vi "Main myRIO.vi"() -> ()   [LabVIEW 2012]
uses:
  <vilib>/rvi/interface/nirviOpenFPGA/nirviOpenFPGA.xnode
  FPGA Bitfiles/PDMSrobotcode_FPGATarget_AllIOs_I1UhDttAVn8.lvbitx
  FPGA/All IOs.vi
  <vilib>/FPGAPlugInAG/myRIO-1900/niLvFpga_Open_myRIO-1900.vi
  <vilib>/rvi/interface/common/dynamic/niFpgaDynamicAddResources.vi
  <vilib>/rvi/interface/nirviReadWriteControl/nirviReadWriteControl.xnode
  <vilib>/rvi/interface/Simulation/niFpgaSimulationCallBeginRW.vi
  <vilib>/rvi/errors/niLvFpgaAdjustHostInterfaceError.vi
  NiFpgaLv.dll
  <vilib>/Utility/error.llb/Error Cluster From Error Code.vi
  <vilib>/rvi/interface/nirviCloseFPGA/nirviCloseFPGA.xnode
  <vilib>/FPGAPlugInAG/Dynamic/niLvFpga_Close_Dynamic.vi
  <vilib>/myRIO/Instrument Drivers/Utilities/Utilities.lvlib
  <vilib>/Instr/_visa.llb/VISA Configure Serial Port (Instr).vi
  <vilib>/myRIO/Instrument Drivers/Onboard IO/UART/typedef/VISA Configuration.ctl
  <vilib>/myRIO/Instrument Drivers/Onboard IO/UART/UART.lvlib
panel:
  in  "Standalone?":bool
  out "BMP180 Data":string
  out "NMEA sentences":string
  out "Time":string
  in  "time zone":i32
  out "Latitude [deg]":string
  out "Longitude [deg]":string
  out "UTC Time":string
  out "Latitude":string
  out "N/S":string
  out "Longitude":string
  out "E/W":string
  out "Speed over ground [knots]":string
  out "Status":string
  out "Course over ground [degrees]":string
  out "Date [ddmmyy]":string
  out "Mode":string
  in  "Acquire?":bool
  out "Frame Rate":dbl
  out "Image Number":u32
  in  "Capture":bool
  in  "Image Logging path":path
  out "Image":T1(plugin-control)
  in  "Down Button":bool
  in  "Left Button":bool
  out "Distance in cm (US BK)":i16
  out "Distance in cm (US FR)":i16
  out "Distance in cm (US FL)":i16
  out "Error":errorcluster
  out "IR Sensors":T2
  in  "Robotic Arm Controls":T3
  in  "Stop Button":bool
  in  "Right Button":bool caption="Next Button"
  in  "Up Button":bool
  out "Inclination":T4(graph)
  # "LED Brightnesses"
  # "GPS Data"
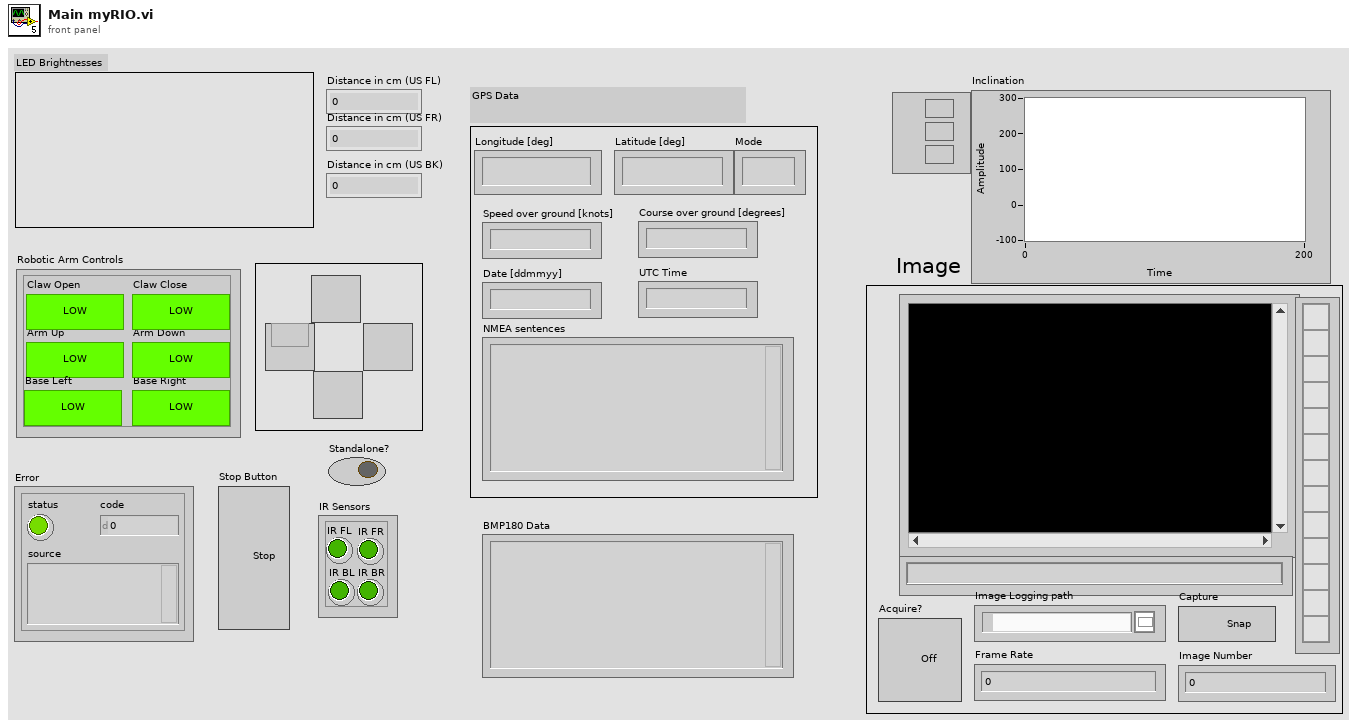
[diagram p1: front panel]
types:
  T1 = typedef "IMAQ Image.ctl" = refnum<image>
  T2 = cluster{"IR FL":bool, "IR FR":bool, "IR BR":bool, "IR BL":bool}
  T3 = cluster{"Arm Up":bool, "Claw Open":bool, "Base Right":bool, "Arm Down":bool, "Base Left":bool, "Claw Close":bool}
  T4 = cluster{"AccelerationX":i16, "AccelerationY":i16, "AccelerationZ":i16}
  T5 = cluster{"Time of flight (uS) (US FL)":u32, "Time of flight (uS) (US FR)":u32, "Time of flight (uS) (US BK)":u32}
  T6 = cluster{"UP":bool, "DOWN":bool, "LEFT":bool, "RIGHT":bool}
  T7 = typedef "UART.lvlib/VISA Configuration.ctl" = cluster{"baud rate (9600)":u32, "data bits (8)":u16, "parity (0:none)":enum16{"None", "Odd", "Even", "Mark", "Space"}, "stop bits (10: 1 bit)":u16, "flow control (0:none)":u16, "termination char\n(0xA = '\\n' = LF) ":u8, "Enable Termination\nChar (T)":bool, "timeout (10sec)":u32}
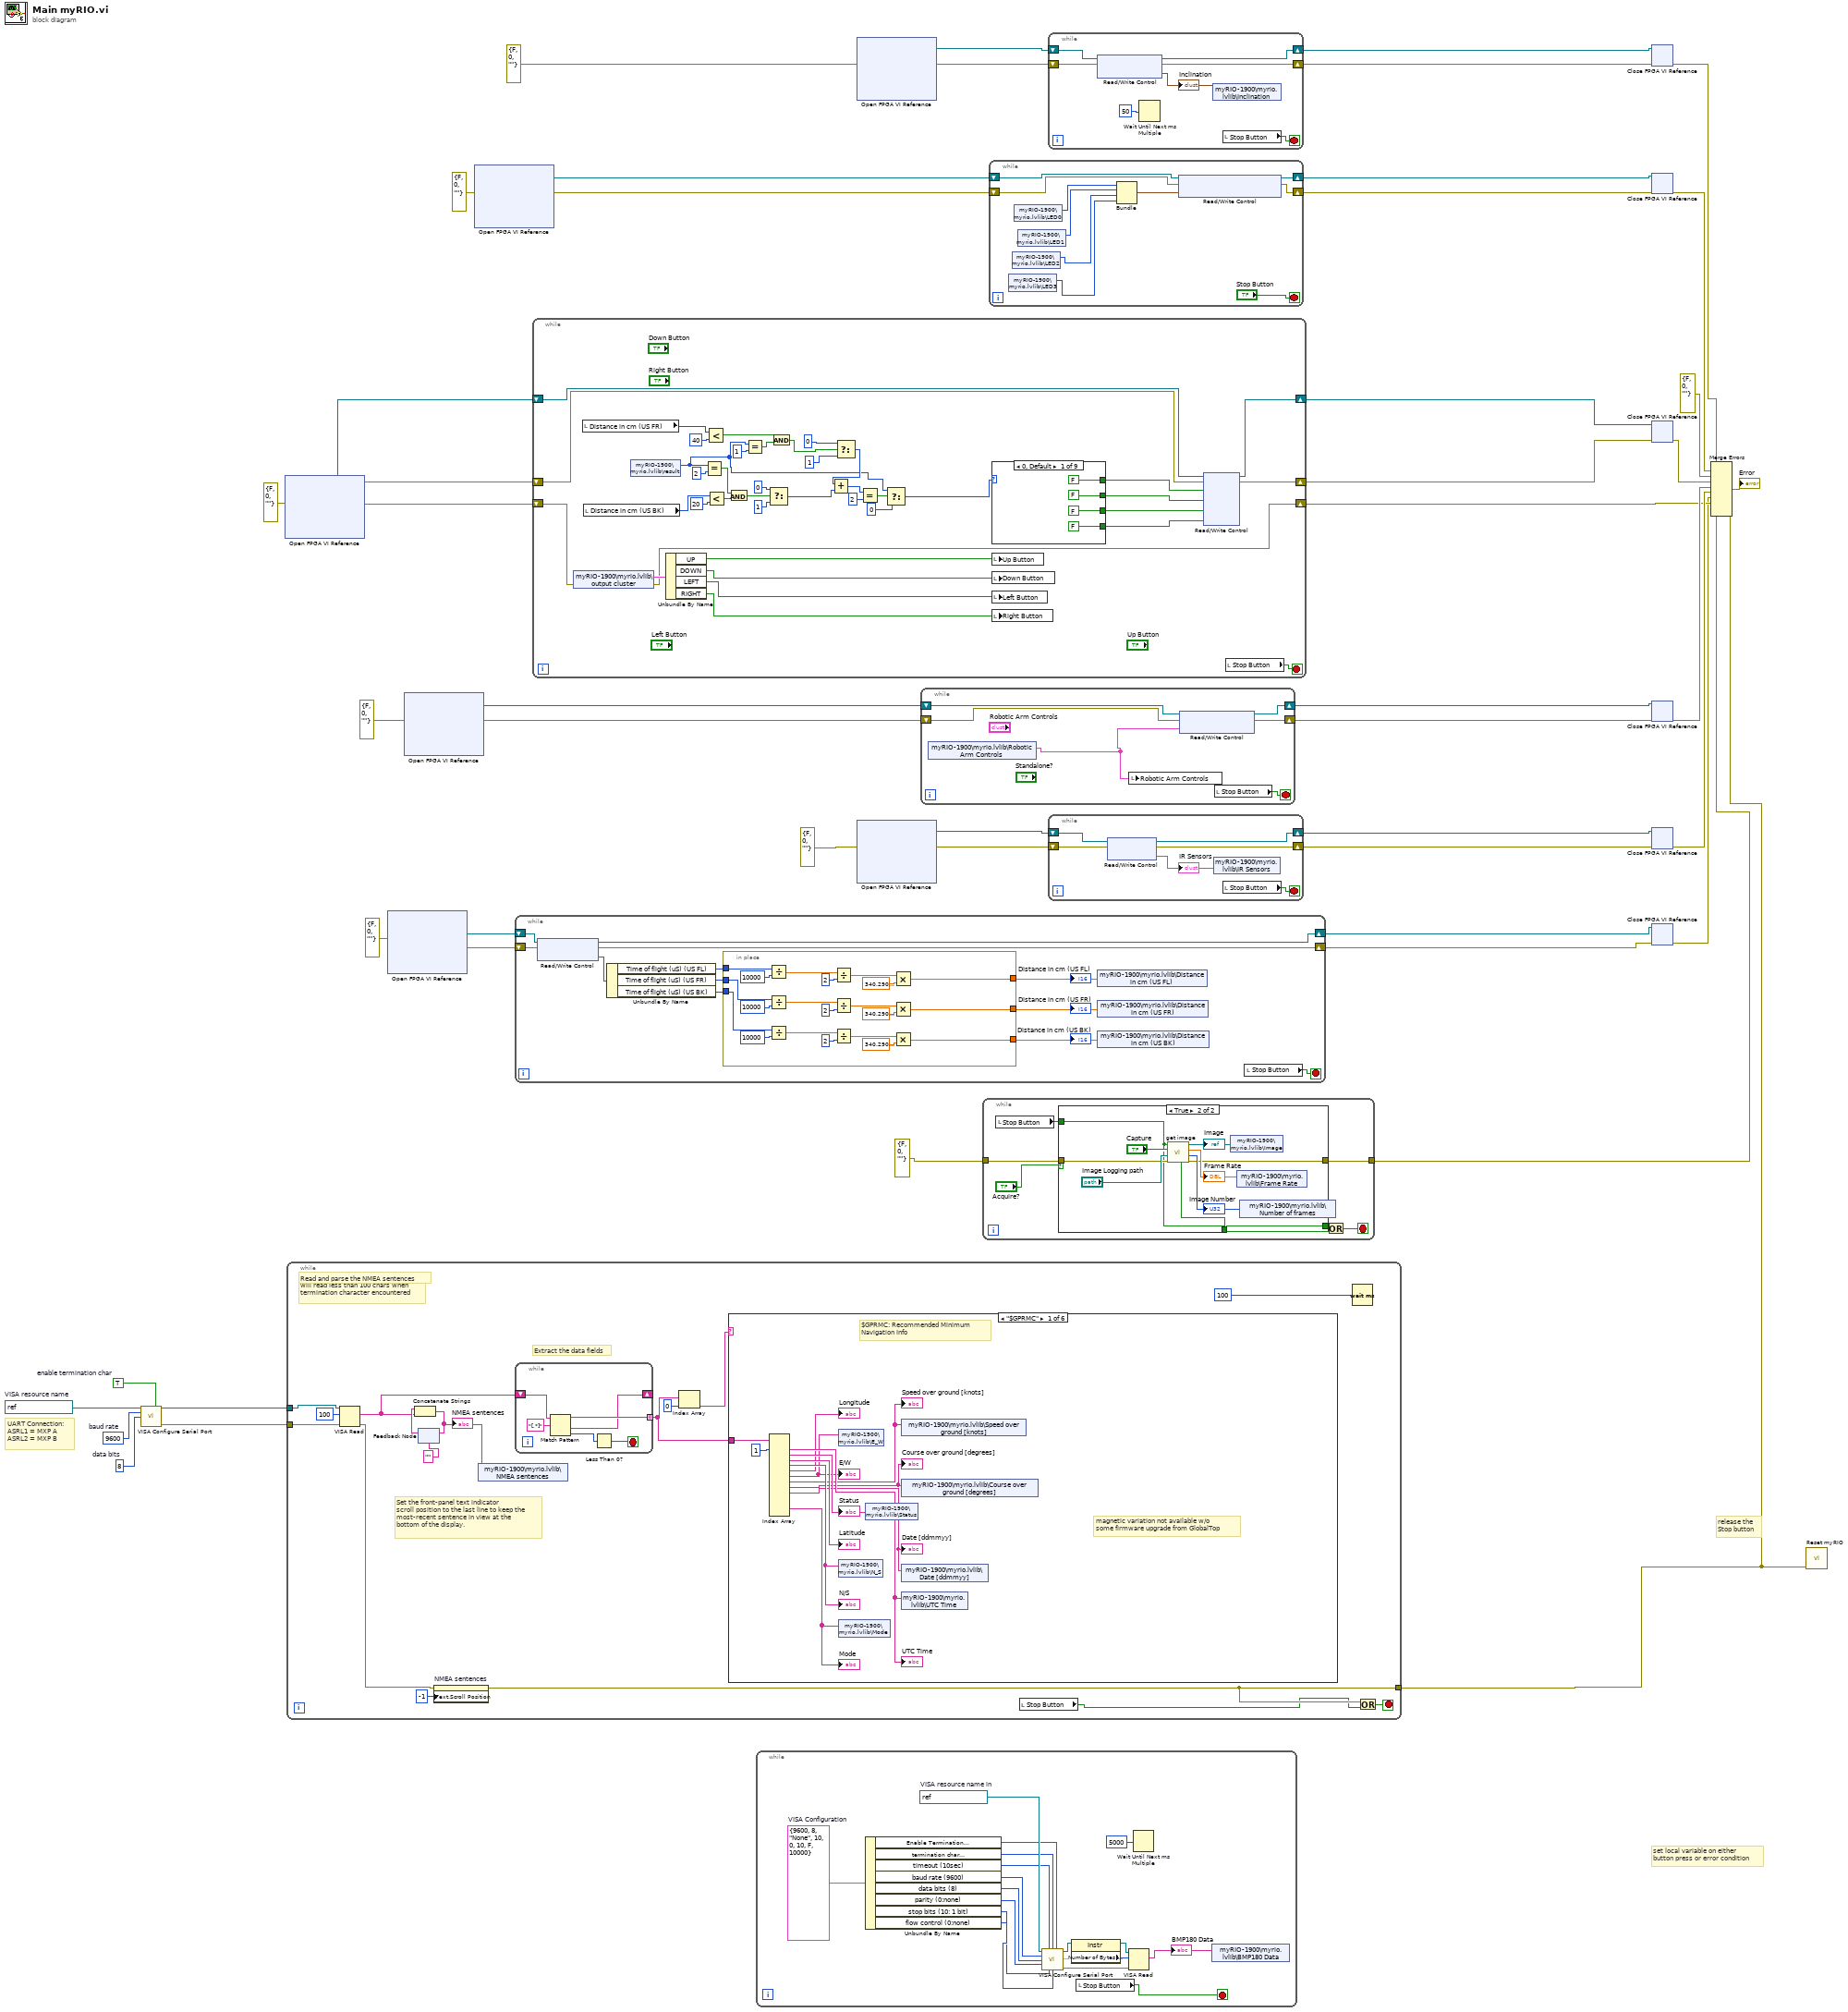
[diagram p0: block diagram]
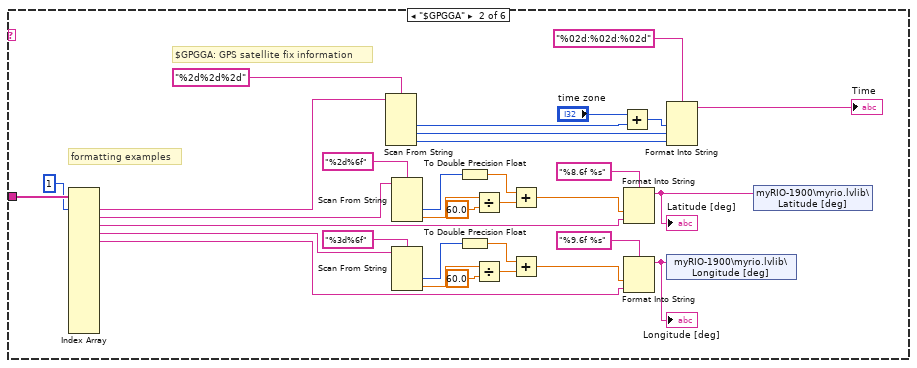
[diagram p2: hidden frame]
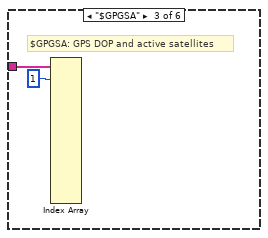
[diagram p3: hidden frame]
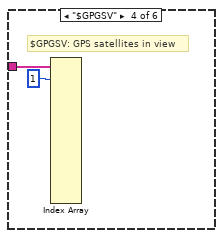
[diagram p4: hidden frame]
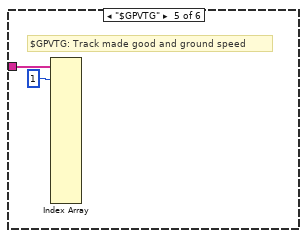
[diagram p5: hidden frame]
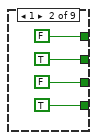
[diagram p8: hidden frame]
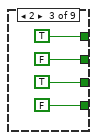
[diagram p9: hidden frame]
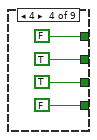
[diagram p10: hidden frame]
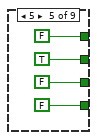
[diagram p11: hidden frame]
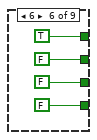
[diagram p12: hidden frame]
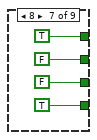
[diagram p13: hidden frame]
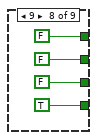
[diagram p14: hidden frame]
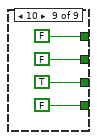
[diagram p15: hidden frame]
diagram:
  w4 = TRUE  # enable termination char
  w5 = u16 8  # data bits
  w6 = u32 9600  # baud rate
  w8 = refnum<visa-resource-name> "ASRL2::INSTR"  # VISA resource name
  # "release the\nStop button"
  # "set local variable on either\nbutton press or error condition"
  # "UART Connection:\nASRL1 = MXP A \nASRL2 = MXP B"
  n1 = call-poly "VISA Configure Serial Port"("VISA resource name"=w8, "Enable Termination\nChar (T)"=w4, "baud rate (9600)"=w6, "data bits (8)"=w5) -> ("VISA resource name out"=w7:refnum<visa-resource-name>, "error out"=w3:errorcluster)  [unwired: 10 in]
  n2 = xnode "Open FPGA VI Reference"("error in"=errorcluster {"status"=FALSE, "code"=0, "source"=""}) -> ("FPGA VI Reference Out"=w35:refnum<k20>, "error out"=w14:errorcluster)  [unwired: 1 in]
  n3 = while {
    tunnel: [w51] -> w2
    tunnel: w7 -> [w63]
    tunnel: w3 -> [w57]
    stop <- w50 stop-if-true
    # "Set the front-panel text indicator\nscroll position to the last line to keep the\nmost-recent sentence in view at the\nbottom of the display."
    # "Read and parse the NMEA sentences"
    # "Extract the data fields"
    # "Read a complete sentence;\nwill read less than 100 chars when\ntermination character encountered"
    n4 = VISA Read(VISA resource name=w63, byte count=u32 100, error in (no error)=w57) -> (read buffer=w58:string, error out=w52:errorcluster)  [unwired: 2 out]
    n5 = feedback #1("") -> (w60:string)
    n6 = Concatenate Strings "Concatenate Strings"(w60, w58) -> (w62:string)
    "NMEA sentences" <- w62
    n7 = feedback-in #1(w62) -> ()
    n8 = property on="NMEA sentences" class="Str"(error in=w52, "Text.Scroll Position"=-1) -> (error out=w51:errorcluster)  [unwired: 1 in, 1 out]
    n9 = shared-variable "myRIO-1900\\myrio.lvlib\\NMEA sentences"(w62) -> ()  [unwired: 1 in, 1 out]
    n10 = while {
      tunnel: [w119] -> w55 mode=indexing
      shift-right: [w118] -> _
      shift-left: w58 -> [w120]
      stop <- w117 stop-if-true
      n11 = Match Pattern(string=w120, regular expression="[,*]") -> (before substring=w119:string, after substring=w118:string, offset past match=w116:i32)  [unwired: 1 in, 1 out]
      n12 = Less Than 0?(x=w116) -> (x < 0?=w117:bool)
    }
    n13 = Index Array "Index Array"(array=w55, index=0) -> (element=w56:string)
    n14 = case shown="\"$GPRMC\"" w56 {
      tunnel: w55 -> [w76 w109 w111 w113 w115 _]
      frame "$GPRMC" {
        # "magnetic variation not available w/o\nsome firmware upgrade from GlobalTop"
        # "$GPRMC: Recommended Minimum\nNavigation Info"
        n15 = Index Array "Index Array"(array=w76, index #1=1 ("index")) -> (element #1=w75:string, element #2=w73:string, element #3=→"Latitude":string, element #4=w71:string, element #5=→"Longitude":string, element #6=w69:string, element #7=w67:string, element #8=w65:string, element #9=w66:string, element #12=w68:string)  [unwired: 12 in, 3 out]
        "UTC Time" <- w75
        "N/S" <- w71
        "E/W" <- w69
        "Speed over ground [knots]" <- w67
        "Status" <- w73
        "Course over ground [degrees]" <- w65
        "Date [ddmmyy]" <- w66
        "Mode" <- w68
        n16 = shared-variable "myRIO-1900\\myrio.lvlib\\E_W"(w69) -> ()  [unwired: 1 in, 1 out]
        n17 = shared-variable "myRIO-1900\\myrio.lvlib\\N_S"(w71) -> ()  [unwired: 1 in, 1 out]
        n18 = shared-variable "myRIO-1900\\myrio.lvlib\\Mode"(w68) -> ()  [unwired: 1 in, 1 out]
        n19 = shared-variable "myRIO-1900\\myrio.lvlib\\Status"(w73) -> ()  [unwired: 1 in, 1 out]
        n20 = shared-variable "myRIO-1900\\myrio.lvlib\\Speed over ground [knots]"(w67) -> ()  [unwired: 1 in, 1 out]
        n21 = shared-variable "myRIO-1900\\myrio.lvlib\\Course over ground [degrees]"(w65) -> ()  [unwired: 1 in, 1 out]
        n22 = shared-variable "myRIO-1900\\myrio.lvlib\\Date [ddmmyy]"(w66) -> ()  [unwired: 1 in, 1 out]
        n23 = shared-variable "myRIO-1900\\myrio.lvlib\\UTC Time"(w75) -> ()  [unwired: 1 in, 1 out]
      }
      frame "$GPGGA" {
        # "formatting examples"
        # "$GPGGA: GPS satellite fix information"
        n24 = Index Array "Index Array"(array=w109, index #1=1 ("index")) -> (element #1=w106:string, element #2=w97:string, element #3=w89:string, element #4=w78:string, element #5=w77:string)  [unwired: 15 in, 11 out]
        n25 = Scan From String "Scan From String"(format string="%2d%2d%2d", input string=w106) -> (output 1=w99:i32, output 2=w102:i32, output 3=w104:i32)  [unwired: 5 in, 3 out]
        n26 = Scan From String(format string="%2d%6f", input string=w97) -> (output 1=w94:i32, output 2=w96:dbl)  [unwired: 4 in, 3 out]
        n27 = Scan From String(format string="%3d%6f", input string=w78) -> (output 1=w82:i32, output 2=w80:dbl)  [unwired: 4 in, 3 out]
        n28 = To Double Precision Float(number=w94) -> (double precision float=w92:dbl)
        n29 = To Double Precision Float(number=w82) -> (double precision float=w84:dbl)
        n30 = Divide(x=w96, y=60.0) -> (x/y=w93:dbl)
        n31 = Divide(x=w80, y=60.0) -> (x/y=w83:dbl)
        n32 = Add(x=w92, y=w93) -> (x+y=w90:dbl)
        n33 = Add(x=w84, y=w83) -> (x+y=w86:dbl)
        n34 = Add(x="time zone", y=w99) -> (x+y=w100:i32)
        n35 = Format Into String(format string="%8.6f %s", w90, w89) -> (resulting string=w88:string)  [unwired: 2 in, 1 out]
        "Latitude [deg]" <- w88
        n36 = Format Into String(format string="%9.6f %s", w86, w77) -> (resulting string=w87:string)  [unwired: 2 in, 1 out]
        "Longitude [deg]" <- w87
        n37 = Format Into String "Format Into String"(format string="%02d:%02d:%02d", w100, w102, w104) -> (resulting string=→"Time":string)  [unwired: 2 in, 1 out]
        n38 = shared-variable "myRIO-1900\\myrio.lvlib\\Longitude [deg]"(w87) -> ()  [unwired: 1 in, 1 out]
        n39 = shared-variable "myRIO-1900\\myrio.lvlib\\Latitude [deg]"(w88) -> ()  [unwired: 1 in, 1 out]
      }
      frame "$GPGSA" {
        # "$GPGSA: GPS DOP and active satellites"
        n40 = Index Array(array=w111, index #1=1 ("index")) -> ()  [unwired: 15 in, 16 out]
      }
      frame "$GPGSV" {
        # "$GPGSV: GPS satellites in view"
        n41 = Index Array(array=w113, index #1=1 ("index")) -> ()  [unwired: 15 in, 16 out]
      }
      frame "$GPVTG" {
        # "$GPVTG: Track made good and ground speed"
        n42 = Index Array(array=w115, index #1=1 ("index")) -> ()  [unwired: 15 in, 16 out]
      }
      frame Default {
      }
    }
    n43 = local read "Stop Button"() -> (w49:bool)
    n44 = Wait (ms)(milliseconds to wait=u32 100) -> ()  [unwired: 1 out]
    n45 = Or(x=w51, y=w49) -> (x .or. y?=w50:bool)
  }
  n46 = xnode "Open FPGA VI Reference"("error in"=errorcluster {"status"=FALSE, "code"=0, "source"=""}) -> ("FPGA VI Reference Out"=w18:refnum<k20>, "error out"=w1:errorcluster)  [unwired: 1 in]
  n47 = xnode "Open FPGA VI Reference"("error in"=errorcluster {"status"=FALSE, "code"=0, "source"=""}) -> ("FPGA VI Reference Out"=w33:refnum<k20>, "error out"=w34:errorcluster)  [unwired: 1 in]
  n48 = xnode "Open FPGA VI Reference"("error in"=errorcluster {"status"=FALSE, "code"=0, "source"=""}) -> ("FPGA VI Reference Out"=w47:refnum<k20>, "error out"=w46:errorcluster)  [unwired: 1 in]
  n49 = while {
    shift-right: [w133] -> w16
    shift-left: w18 -> [w131]
    shift-right: [w132] -> w17
    shift-left: w1 -> [w130]
    stop <- w129 stop-if-true
    n50 = xnode "Read/Write Control"("FPGA VI Reference In"=w131, "error in"=w130) -> ("FPGA VI Reference Out"=w133:refnum<k20>, "error out"=w132:errorcluster, "Time of flight"=w128:T5)
    n51 = Unbundle By Name(w128) -> ("Time of flight (uS) (US FL)"=w127:u32, "Time of flight (uS) (US FR)"=w126:u32, "Time of flight (uS) (US BK)"=w125:u32)
    n52 = in-place {
      in-place-border: w127 -> [w139]
      in-place-border: w126 -> [w138]
      in-place-border: w125 -> [w137]
      in-place-border: [w136] -> w124
      in-place-border: [w135] -> w123
      in-place-border: [w134] -> w122
      n53 = Divide(x=w139, y=u32 10000) -> (x/y=w153:sgl)
      n54 = Divide(x=w138, y=u32 10000) -> (x/y=w146:sgl)
      n55 = Divide(x=w137, y=u32 10000) -> (x/y=w143:sgl)
      n56 = Divide(x=w153, y=u8 2) -> (x/y=w152:sgl)
      n57 = Divide(x=w146, y=u8 2) -> (x/y=w147:sgl)
      n58 = Divide(x=w143, y=u8 2) -> (x/y=w142:sgl)
      n59 = Multiply(x=w152, y=sgl 340.29) -> (x*y=w134:sgl)
      n60 = Multiply(x=w147, y=sgl 340.29) -> (x*y=w135:sgl)
      n61 = Multiply(x=w142, y=sgl 340.29) -> (x*y=w136:sgl)
    }
    "Distance in cm (US FL)" <- w122
    "Distance in cm (US FR)" <- w123
    "Distance in cm (US BK)" <- w124
    n62 = shared-variable "myRIO-1900\\myrio.lvlib\\Distance in cm (US FL)"(w122) -> ()  [unwired: 1 in, 1 out]
    n63 = shared-variable "myRIO-1900\\myrio.lvlib\\Distance in cm (US FR)"(w123) -> ()  [unwired: 1 in, 1 out]
    n64 = shared-variable "myRIO-1900\\myrio.lvlib\\Distance in cm (US BK)"(w124) -> ()  [unwired: 1 in, 1 out]
    n65 = local read "Stop Button"() -> (w129:bool)
  }
  n66 = while {
    shift-right: [w194] -> w37
    shift-left: w35 -> [w192]
    shift-right: [w193] -> w36
    shift-left: w14 -> [w191]
    shift-right: [w179] -> w13
    shift-left: w14 -> [w180]
    stop <- w190 stop-if-true
    n67 = shared-variable "myRIO-1900\\myrio.lvlib\\output cluster"(error in=w180) -> (w181:T6, error out=w179:errorcluster)
    n68 = local read "Distance in cm (US FR)"() -> (w170:i16)
    n69 = local read "Distance in cm (US BK)"() -> (w177:i16)
    n70 = shared-variable "myRIO-1900\\myrio.lvlib\\result"() -> (w157:i32)  [unwired: 1 in, 1 out]
    n71 = Unbundle By Name(w181) -> ("UP"=w189:bool, "DOWN"=w188:bool, "LEFT"=w187:bool, "RIGHT"=w186:bool)
    n72 = Equal?(x=w157, y=2) -> (x = y?=w173:bool)
    n73 = Less?(x=w170, y=40) -> (x < y?=w167:bool)
    n74 = Less?(x=w177, y=20) -> (x < y?=w174:bool)
    n75 = And(x=w173, y=w174) -> (x .and. y?=w172:bool)
    n76 = Equal?(x=w157, y=1) -> (x = y?=w168:bool)
    n77 = Select(t=0, s=w172, f=1) -> (s? t:f=w162:i32)
    n78 = And(x=w167, y=w168) -> (x .and. y?=w165:bool)
    n79 = Select(t=0, s=w165, f=1) -> (s? t:f=w161:i32)
    n80 = Add(x=w161, y=w162) -> (x+y=w160:i32)
    n81 = Equal?(x=w160, y=2) -> (x = y?=w158:bool)
    n82 = Select(t=w157, s=w158, f=0) -> (s? t:f=w155:i32)
    n83 = case shown="0, Default" w155 {
      tunnel: [FALSE FALSE TRUE FALSE FALSE TRUE TRUE FALSE FALSE] -> w185
      tunnel: [FALSE TRUE FALSE TRUE TRUE FALSE FALSE FALSE FALSE] -> w184
      tunnel: [FALSE FALSE TRUE TRUE FALSE FALSE FALSE FALSE TRUE] -> w183
      tunnel: [FALSE TRUE FALSE FALSE FALSE FALSE TRUE TRUE FALSE] -> w182
      frame 0, Default {
      }
      frame 1 {
      }
      frame 2 {
      }
      frame 4 {
      }
      frame 5 {
      }
      frame 6 {
      }
      frame 8 {
      }
      frame 9 {
      }
      frame 10 {
      }
    }
    n84 = local write "Up Button"(w189) -> ()
    n85 = local write "Down Button"(w188) -> ()
    n86 = local write "Left Button"(w187) -> ()
    n87 = local write "Right Button"(w186) -> ()
    n88 = xnode "Read/Write Control"("FPGA VI Reference In"=w192, "error in"=w191, "BR"=w185, "FR"=w184, "BL"=w183, "FL"=w182) -> ("FPGA VI Reference Out"=w194:refnum<k20>, "error out"=w193:errorcluster)
    n89 = local read "Stop Button"() -> (w190:bool)
  }
  n90 = while {
    stop <- w233 stop-if-true
    w246 = T7 {"baud rate (9600)"=9600, "data bits (8)"=8, "parity (0:none)"=enum."None", "stop bits (10: 1 bit)"=10, "flow control (0:none)"=0, "termination char\n(0xA = '\\n' = LF) "=10, "Enable Termination\nChar (T)"=FALSE, "timeout (10sec)"=10000}  # VISA Configuration
    w247 = refnum<visa-resource-name> "ASRL1::INSTR"  # VISA resource name in
    n91 = Unbundle By Name(w246) -> ("Enable Termination\nChar (T)"=w243:bool, "termination char\n(0xA = '\\n' = LF)"=w242:u8, "timeout (10sec)"=w241:u32, "baud rate (9600)"=w236:u32, "data bits (8)"=w237:u16, "parity (0:none)"=w238:enum16{"None", "Odd", "Even", "Mark", "Space"}, "stop bits (10: 1 bit)"=w239:u16, "flow control (0:none)"=w240:u16)
    n92 = call-poly "VISA Configure Serial Port"("VISA resource name"=w247, "timeout (10sec)"=w241, "termination char\n(0xA = '\\n' = LF)"=w242, "Enable Termination\nChar (T)"=w243, "baud rate (9600)"=w236, "data bits (8)"=w237, "parity (0:none)"=w238, "stop bits (10: 1 bit)"=w239, "flow control (0:none)"=w240) -> ("VISA resource name out"=w245:refnum<visa-resource-name>, "error out"=w244:errorcluster)  [unwired: 5 in]
    n93 = property class="Instr"(reference=w245) -> (reference out=w234:refnum<visa-resource-name>, "Serial Settings:Number of Bytes at Serial Port"=w235:u32)  [unwired: 1 in, 1 out]
    n94 = local read "Stop Button"() -> (w233:bool)
    n95 = VISA Read(VISA resource name=w234, byte count=w235, error in (no error)=w244) -> (read buffer=w232:string)  [unwired: 3 out]
    "BMP180 Data" <- w232
    n96 = Wait Until Next ms Multiple(millisecond multiple=u32 5000) -> ()  [unwired: 1 out]
    n97 = shared-variable "myRIO-1900\\myrio.lvlib\\BMP180 Data"(w232) -> ()  [unwired: 1 in, 1 out]
  }
  n98 = xnode "Open FPGA VI Reference"("error in"=errorcluster {"status"=FALSE, "code"=0, "source"=""}) -> ("FPGA VI Reference Out"=w42:refnum<k20>, "error out"=w41:errorcluster)  [unwired: 1 in]
  n99 = xnode "Open FPGA VI Reference"("error in"=errorcluster {"status"=FALSE, "code"=0, "source"=""}) -> ("FPGA VI Reference Out"=w26:refnum<k20>, "error out"=w25:errorcluster)  [unwired: 1 in]
  n100 = while {
    shift-right: [w253] -> w31
    shift-left: w33 -> [w251]
    shift-right: [w252] -> w32
    shift-left: w34 -> [w250]
    stop <- w249 stop-if-true
    n101 = shared-variable "myRIO-1900\\myrio.lvlib\\Robotic Arm Controls"() -> (w248:T3)  [unwired: 1 in, 1 out]
    n102 = local write "Robotic Arm Controls"(w248) -> ()
    n103 = xnode "Read/Write Control"("FPGA VI Reference In"=w251, "error in"=w250, "Robotic Arm I/Os"=w248) -> ("FPGA VI Reference Out"=w253:refnum<k20>, "error out"=w252:errorcluster)
    n104 = local read "Stop Button"() -> (w249:bool)
  }
  n105 = while {
    tunnel: errorcluster {"status"=FALSE, "code"=0, "source"=""} ("error constant") -> [w257]
    tunnel: [w256] -> w9
    stop <- w258 stop-if-true
    n106 = local read "Stop Button"() -> (w254:bool)
    n107 = case shown="True" "Acquire?" {
      tunnel: [_ w263] -> w260
      tunnel: [w261 w266] -> w259
      tunnel: w257 -> [w262 w265]
      tunnel: [w262 w264] -> w256
      tunnel: w254 -> [w261 w263]
      frame False {
      }
      frame True {
        n108 = call "get image.vi"("error in"=w265, "Image Logging Path"="Image Logging path", "Log Image"="Capture", "Stop (F)"=w263) -> ("error out"=w264:errorcluster, "Image Number"=w268:u32, "Frame Rate"=w267:dbl, "Image Out"=w271:T1, "Stopped"=w266:bool)  [unwired: 3 in]
        "Image" <- w271
        "Image Number" <- w268
        "Frame Rate" <- w267
        n109 = shared-variable "myRIO-1900\\myrio.lvlib\\Image"(w271) -> ()  [unwired: 1 in, 1 out]
        n110 = shared-variable "myRIO-1900\\myrio.lvlib\\Frame Rate"(w267) -> ()  [unwired: 1 in, 1 out]
        n111 = shared-variable "myRIO-1900\\myrio.lvlib\\Number of frames"(w268) -> ()  [unwired: 1 in, 1 out]
      }
    }
    n112 = Or(x=w260, y=w259) -> (x .or. y?=w258:bool)
  }
  n113 = while {
    shift-right: [w279] -> w45
    shift-left: w47 -> [w281]
    shift-right: [w278] -> w44
    shift-left: w46 -> [w280]
    stop <- "Stop Button" stop-if-true
    n114 = shared-variable "myRIO-1900\\myrio.lvlib\\LED3"() -> (w276:u8)  [unwired: 1 in, 1 out]
    n115 = shared-variable "myRIO-1900\\myrio.lvlib\\LED2"() -> (w275:u8)  [unwired: 1 in, 1 out]
    n116 = shared-variable "myRIO-1900\\myrio.lvlib\\LED0"() -> (w274:u8)  [unwired: 1 in, 1 out]
    n117 = shared-variable "myRIO-1900\\myrio.lvlib\\LED1"() -> (w273:u8)  [unwired: 1 in, 1 out]
    n118 = Bundle(w274, w273, w275, w276) -> (w272:cluster{u8, u8, u8, u8})  [unwired: 1 in]
    n119 = xnode "Read/Write Control"("FPGA VI Reference In"=w281, "error in"=w280, "On-board LED Brightness"=w272) -> ("FPGA VI Reference Out"=w279:refnum<k20>, "error out"=w278:errorcluster)
  }
  n120 = while {
    shift-right: [w284] -> w40
    shift-left: w42 -> [w288]
    shift-right: [w283] -> w39
    shift-left: w41 -> [w287]
    stop <- w285 stop-if-true
    n121 = xnode "Read/Write Control"("FPGA VI Reference In"=w288, "error in"=w287) -> ("FPGA VI Reference Out"=w284:refnum<k20>, "error out"=w283:errorcluster, "Accelerometer"=w286:T4)
    "Inclination" <- w286
    n122 = Wait Until Next ms Multiple(millisecond multiple=u32 50) -> ()  [unwired: 1 out]
    n123 = shared-variable "myRIO-1900\\myrio.lvlib\\Inclination"(w286) -> ()  [unwired: 1 in, 1 out]
    n124 = local read "Stop Button"() -> (w285:bool)
  }
  n125 = while {
    shift-right: [w294] -> w28
    shift-left: w26 -> [w292]
    shift-right: [w293] -> w27
    shift-left: w25 -> [w291]
    stop <- w289 stop-if-true
    n126 = xnode "Read/Write Control"("FPGA VI Reference In"=w292, "error in"=w291) -> ("FPGA VI Reference Out"=w294:refnum<k20>, "error out"=w293:errorcluster, "IR Sensors"=w290)
    "IR Sensors" <- w290
    n127 = shared-variable "myRIO-1900\\myrio.lvlib\\IR Sensors"(w290) -> ()  [unwired: 1 in, 1 out]
    n128 = local read "Stop Button"() -> (w289:bool)
  }
  n129 = xnode "Close FPGA VI Reference"("FPGA VI Reference In"=w40, "error in"=w39) -> ("error out"=w24:errorcluster)
  n130 = xnode "Close FPGA VI Reference"("FPGA VI Reference In"=w45, "error in"=w44) -> ("error out"=w23:errorcluster)
  n131 = xnode "Close FPGA VI Reference"("FPGA VI Reference In"=w37, "error in"=w36) -> ("error out"=w22:errorcluster)
  n132 = xnode "Close FPGA VI Reference"("FPGA VI Reference In"=w31, "error in"=w32) -> ("error out"=w21:errorcluster)
  n133 = xnode "Close FPGA VI Reference"("FPGA VI Reference In"=w28, "error in"=w27) -> ("error out"=w20:errorcluster)
  n134 = xnode "Close FPGA VI Reference"("FPGA VI Reference In"=w16, "error in"=w17) -> ("error out"=w10:errorcluster)
  n135 = Merge Errors(w24, w23, errorcluster {"status"=FALSE, "code"=0, "source"=""} ("error in"), w22, w21, w20, w10, w13, w9, w2) -> (→"Error":errorcluster)
  n136 = call <vilib>:"Reset myRIO.vi"("error in (no error)"=w2) -> ()  [unwired: 10 in, 1 out]
